vi "AIDecode.vi"(11 "String":string) -> (2 "AIData":dbl[](array[numeric]), 3 "AIChannels":u8[](array[numeric]))   [LabVIEW 2017]
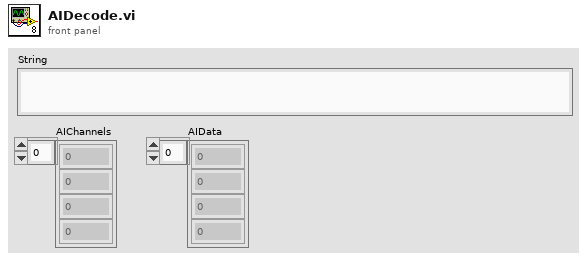
[diagram p1: front panel]
types:
  T1 = cluster{"String":string, "String":string, "String":string}
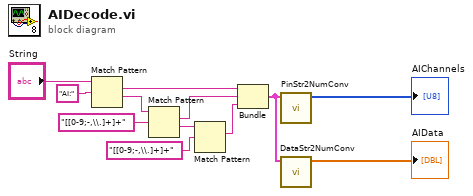
[diagram p0: block diagram]
diagram:
  n1 = Match Pattern(string="String", regular expression="AI:") -> (match substring=w6:string, after substring=w10:string)  [unwired: 1 in, 2 out]
  n2 = Match Pattern(string=w10, regular expression="[[0-9;-,\\.]+]+") -> (match substring=w4:string, after substring=w7:string)  [unwired: 1 in, 2 out]
  n3 = Match Pattern(string=w7, regular expression="[[0-9;-,\\.]+]+") -> (match substring=w5:string)  [unwired: 1 in, 3 out]
  n4 = Bundle("String"=w6, "String"=w4, "String"=w5) -> (w3:T1)  [unwired: 1 in]
  n5 = call "PinStr2NumConv.vi"("Cluster"=w3) -> ("Array"=→"AIChannels":u8[])  [unwired: 10 in]
  n6 = call "DataStr2NumConv.vi"("Cluster"=w3) -> ("Array"=→"AIData":dbl[])  [unwired: 10 in]
